vi "PH_Beckhoff_PP_PU.set Ignitron GUI Elements to Default.vi"(0 "i ref in":refnum<vi>, 2 "PUs":T2[](array[typedef]), 5 "error in":errorcluster) -> (14 "i ref out":refnum<vi>, 19 "error out":errorcluster)   [LabVIEW 2014, in "PH_Beckhoff_PP_PU.lvlib"]
uses:
  PH_Beckhoff_PP_PU.lvlib
  PH_PP_Common/PH_PP_Common.PUs.ctl
  PH_Beckhoff_PP_PU.Igni Tags.ctl
  PH_Common/Names/PH_Names.Subsystems.ctl
  PH_PP_Common/PH_PP_Common.Devices.ctl
  PH_Common/PH_Common.lvlib
  PH_PP_Common/PH_PP_Common.lvlib
panel:
  in  "Ignitron Tags":T1
  in  "PU":T2
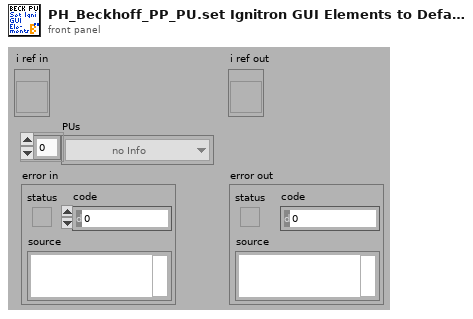
[diagram p1: front panel]
types:
  T1 = typedef "PH_Beckhoff_PP_PU.lvlib/PH_Beckhoff_PP_PU.Igni Tags.ctl" = enum16{"heating-on", "water-on", "Device-on", "Status"}
  T2 = typedef "PH_PP_Common.lvlib/PH_PP_Common.PUs.ctl" = enum16{"no Info", "PA-19mm-1", "PA-19mm-2", "PA-45mm-PILC", "PA-45mm-MAIN", "MA-PU-1", "MA-PU-2", "MA-PU-3", "MA-PU-4", "MA-PU-5", "MA-PU-6", "MA-FR", "MA-PILC", "PA-45mm-DP"}
  T3 = typedef "PH_Common.lvlib/PH_Names.Subsystems.ctl" = enum16{"no Info", "fs-FE", "ns-FE", "PA", "MA", "MAS", "COS", "Exp-LB", "Exp-LL", "PP", "PILS"}
  T4 = typedef "PH_Beckhoff_PP_PU.lvlib/PH_Beckhoff_PP_PU.i attribute.ctl" = cluster{"HV Meas":cluster{"Input GUI Ref":refnum<vi>, "Voltage Service ID":i32, "Voltage [V]":dbl, "Quality":bool, "# in Data":i32}[], "Trigger":cluster{"Status":cluster{"GUI Ref":refnum<vi>, "Status Service ID":i32, "Status":T5}, "last shot:":cluster{"GUI Ref":refnum<vi>, "Service ID":i32, "Time":string}, "DIs":cluster{"triggered":cluster{"GUI Ref":refnum<vi>, "# in Data":i32}, "fired":cluster{"GUI Ref":refnum<vi>, "# in Data":i32}}, "GUI Ref Indicator":refnum<vi>}[], "RR":cluster{"Status":cluster{"GUI Ref":refnum<vi>, "Status Service ID":i32, "Status":T5}, "DIs":cluster{"closed":cluster{"GUI Ref":refnum<vi>, "# in Data":i32}, "open":cluster{"GUI Ref":refnum<vi>, "# in Data":i32}}, "Close":cluster{"GUI Ref":refnum<vi>, "# in Data":i32}, "GUI Ref Indicator":refnum<vi>}[], "Igni":cluster{"Status":cluster{"GUI Ref":refnum<vi>, "Status Service ID":i32, "Status":T5}, "DIs":cluster{"heating on":cluster{"GUI Ref":refnum<vi>, "# in Data":i32}, "water on":cluster{"GUI Ref":refnum<vi>, "# in Data":i32}}, "Device on":cluster{"GUI Ref":refnum<vi>, "# in Data":i32}, "GUI Ref Indicator":refnum<vi>}[], "PSU":cluster{"Status":cluster{"GUI Ref":refnum<vi>, "Status Service ID":i32, "Status":T5}, "Limit Service ID":i32, "DIs":cluster{"inhibit":cluster{"GUI Ref":refnum<vi>, "# in Data":i32}, "end of charge":cluster{"GUI Ref":refnum<vi>, "# in Data":i32}, "HV on":cluster{"GUI Ref":refnum<vi>, "# in Data":i32}, "overtemp":cluster{"GUI Ref":refnum<vi>, "# in Data":i32}, "interlock":cluster{"GUI Ref":refnum<vi>, "# in Data":i32}, "load fault":cluster{"GUI Ref":refnum<vi>, "# in Data":i32}, "sum fault":cluster{"GUI Ref":refnum<vi>, "# in Data":i32}, "HV off":cluster{"GUI Ref":refnum<vi>, "# in Data":i32}, "DC ok":cluster{"GUI Ref":refnum<vi>, "# in Data":i32}}, "AIs":cluster{"voltage":cluster{"GUI Ref":refnum<vi>, "# in Data":i32}, "current":cluster{"GUI Ref":refnum<vi>, "# in Data":i32}}, "DAs":cluster{"inhibit":cluster{"GUI Ref":refnum<vi>, "# in Data":i32}, "interlock":cluster{"GUI Ref":refnum<vi>, "# in Data":i32}, "HV on":cluster{"GUI Ref":refnum<vi>, "# in Data":i32}, "Reset":cluster{"GUI Ref":refnum<vi>, "# in Data":i32}}, "AAs":cluster{"Voltage to set":cluster{"GUI Ref":refnum<vi>, "# in Data":i32}}, "GUI Ref Indicator":refnum<vi>}[], "reconfigured":cluster{"?":bool, "GUI Ref":refnum<vi>}, "PU Rack Type":T6, "HV Meas Info":T7, "PSU Info":T8}
  T5 = typedef "PH_StatusHandler.lvlib/PH_StatusHandler.Status.ctl" = i16
  T6 = typedef "PH_Beckhoff_PP_PU.lvlib/PH_Beckhoff_PP_PU.PU Rack Type.ctl" = enum16{"no Info", "PA 19mm", "PA 45mm", "MA PU 1 and 2", "MA PU 3 and 4", "MA PU 5 and 6", "MA FR and PILC"}
  T7 = typedef "PH_Beckhoff_PP_PU.lvlib/PH_Beckhoff_PP_PU.HV Meas Info.ctl" = cluster{"Period Time [s]":dbl, "Subtractor 1 [Hz]":dbl, "Devider 1 [Hz/kV]":dbl, "Subtractor 2 [Hz]":dbl, "Devider 2 [Hz/kV]":dbl}
  T8 = typedef "PH_Beckhoff_PP_PU.lvlib/PH_Beckhoff_PP_PU.PSU Info.ctl" = cluster{"Limits 1 [V]":cluster{"Lower":dbl, "Upper":dbl}, "Limits 2 [V]":cluster{"Lower":dbl, "Upper":dbl}}
  T9 = cluster{"Status":cluster{"GUI Ref":refnum<vi>, "Status Service ID":i32, "Status":T5}, "DIs":cluster{"heating on":cluster{"GUI Ref":refnum<vi>, "# in Data":i32}, "water on":cluster{"GUI Ref":refnum<vi>, "# in Data":i32}}, "Device on":cluster{"GUI Ref":refnum<vi>, "# in Data":i32}, "GUI Ref Indicator":refnum<vi>}[]
  T10 = typedef "PH_PP_Common.lvlib/PH_PP_Common.Devices.ctl" = enum16{"no Info", "Igni", "RR", "DumpRoss", "PSU", "Trigger", "HV-Meas", "Rods", "Chiller", "Conductivity", "Mercury"}
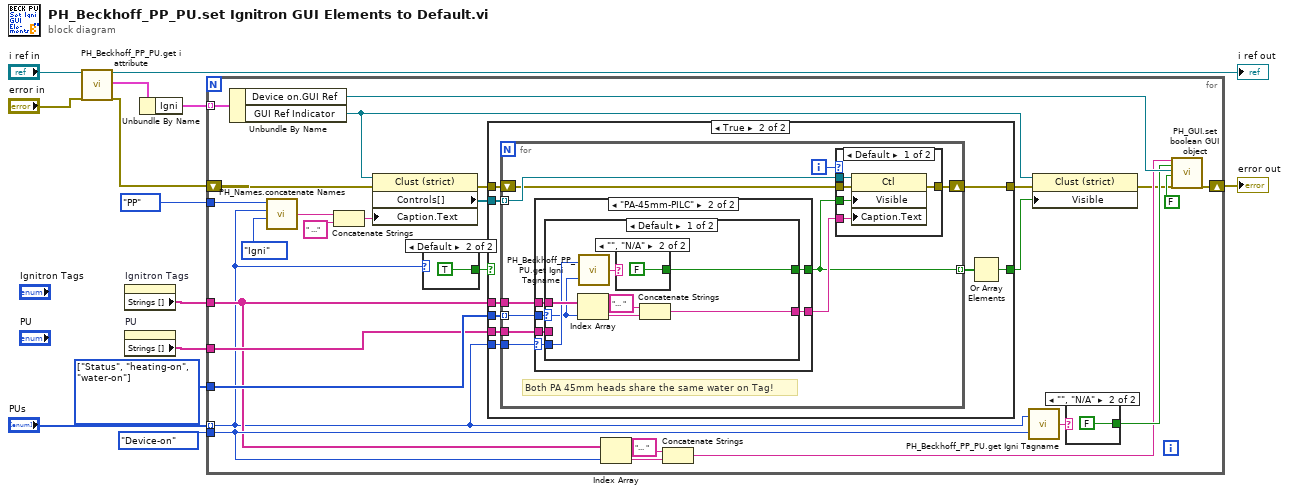
[diagram p0: block diagram]
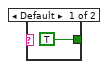
[diagram p2: hidden frame]
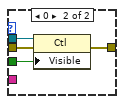
[diagram p4: hidden frame]
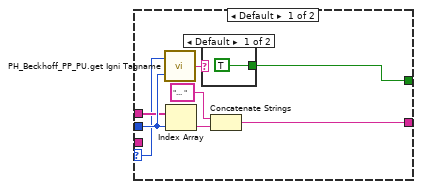
[diagram p5: hidden frame]
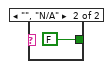
[diagram p6: hidden frame]
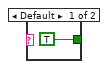
[diagram p7: hidden frame]
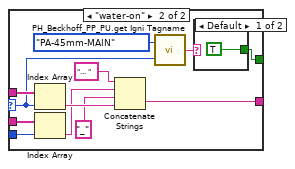
[diagram p8: hidden frame]
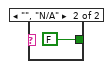
[diagram p9: hidden frame]
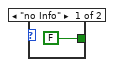
[diagram p10: hidden frame]
diagram:
  w2 = T1[] [enum."Status", enum."heating-on", enum."water-on"] items=["heating-on", "water-on", "Device-on", "Status"]
  n1 = call "PH_Beckhoff_PP_PU.get i attribute.vi"("i ref in"="i ref in", "error in (no error)"="error in") -> ("i ref out"=→"i ref out":refnum<vi>, "i attribute"=w10:T4, "error out"=w8:errorcluster)  [unwired: 15 in]
  n2 = property on="Ignitron Tags" class="Enum (strict)"() -> ("Strings []"=w3:string[])  [unwired: 2 in, 2 out]
  n3 = property on="PU" class="Enum (strict)"() -> ("Strings []"=w11:string[])  [unwired: 2 in, 2 out]
  n4 = Unbundle By Name(w10) -> ("Igni"=w9:T9)
  n5 = for {
    tunnel: w9 -> [w40] mode=indexing
    shift-right: [w32] -> w12
    shift-left: w8 -> [w38]
    tunnel: "PUs" -> [w21] mode=indexing
    tunnel: w2 -> [w37]
    tunnel: w11 -> [w26]
    tunnel: w3 -> [w22]
    tunnel: PH_Beckhoff_PP_PU.Igni_Tags."Device-on" ("Igni Tag") -> [w25]
    tunnel: PH_Names.Subsystems."PP" ("Subsystem") -> [w19]
    n6 = Unbundle By Name(w40) -> ("Device on.GUI Ref"=w31:refnum<vi>, "GUI Ref Indicator"=w15:refnum<vi>)
    n7 = call "PH_Names.concatenate Names.vi"("Devices (no info)"=PH_PP_Common.Devices."Igni", "PU (no info)"=w21, "Subsystem"=w19) -> ("Subsystem_PU_Devices_Comm Type"=w20:string)  [unwired: 1 in]
    n8 = Concatenate Strings(w20, " ..." ("string")) -> (w34:string)
    n9 = property class="Clust (strict)"(reference=w15, error in=w38, "Caption.Text"=w34) -> (error out=w39:errorcluster, "Controls[]"=w35:refnum<vi>[])  [unwired: 1 out]
    n10 = case shown="Default" w21 {
      tunnel: [FALSE TRUE] -> w36
      frame "no Info" {
      }
      frame Default {
      }
    }
    n11 = case shown="True" w36 {
      selector: w36 -> [w43 _]
      tunnel: w35 -> [_ w53]
      tunnel: w39 -> [w44 w52]
      tunnel: [w44 w51] -> w16
      tunnel: w37 -> [_ w50]
      tunnel: w21 -> [_ w49]
      tunnel: w22 -> [_ w48]
      tunnel: w26 -> [_ w47]
      tunnel: [w43 w45] -> w14
      frame False {
      }
      frame True {
        n12 = for {
          tunnel: w53 -> [w56] mode=indexing
          shift-right: [w59] -> w51
          shift-left: w52 -> [w55]
          tunnel: w49 -> [w61]
          tunnel: w50 -> [w63] mode=indexing
          tunnel: w48 -> [w62]
          tunnel: w47 -> [w60]
          tunnel: [w54] -> w46 mode=indexing
          i -> [w57]
          # "Both PA 45mm heads share the same water on Tag!"
          n13 = case shown="\"PA-45mm-PILC\"" w61 {
            selector: w61 -> [w75 w87]
            tunnel: w63 -> [w80 w86]
            tunnel: w62 -> [w79 w88]
            tunnel: w60 -> [_ w85]
            tunnel: [w73 w84] -> w54
            tunnel: [w74 w83] -> w58
            frame Default {
              n14 = call "PH_Beckhoff_PP_PU.get Igni Tagname.vi"("Igni Tag"=w80, "PU"=w75) -> ("Igni Tagname"=w78:string)
              n15 = Index Array(array=w79, index=w80) -> (element=w77:string)
              n16 = case shown="Default" w78 {
                tunnel: [TRUE FALSE] -> w73
                frame Default {
                }
                frame "", "N/A" {
                }
              }
              n17 = Concatenate Strings("... " ("string"), w77) -> (w74:string)
            }
            frame "PA-45mm-PILC" {
              n18 = case shown="Default" w86 {
                selector: w86 -> [w91 w107]
                tunnel: w88 -> [w96 w110]
                tunnel: w87 -> [w92 w102]
                tunnel: w85 -> [_ w101]
                tunnel: [w89 w99] -> w83
                tunnel: [w90 w100] -> w84
                frame Default {
                  n19 = Index Array(array=w96, index=w91) -> (element=w94:string)
                  n20 = call "PH_Beckhoff_PP_PU.get Igni Tagname.vi"("Igni Tag"=w91, "PU"=w92) -> ("Igni Tagname"=w95:string)
                  n21 = case shown="\"\", \"N/A\"" w95 {
                    tunnel: [TRUE FALSE] -> w90
                    frame Default {
                    }
                    frame "", "N/A" {
                    }
                  }
                  n22 = Concatenate Strings("... " ("string"), w94) -> (w89:string)
                }
                frame "water-on" {
                  n23 = Index Array(array=w110, index=w107) -> (element=w108:string)
                  n24 = Index Array(array=w101, index=w102) -> (element=w104:string)
                  n25 = Concatenate Strings("... " ("string"), w104, "_" ("string"), w108) -> (w99:string)
                  n26 = call "PH_Beckhoff_PP_PU.get Igni Tagname.vi"("Igni Tag"=w107, "PU"=PH_PP_Common.PUs."PA-45mm-MAIN") -> ("Igni Tagname"=w109:string)
                  n27 = case shown="Default" w109 {
                    tunnel: [TRUE FALSE] -> w100
                    frame Default {
                    }
                    frame "", "N/A" {
                    }
                  }
                }
              }
            }
          }
          n28 = case shown="Default" w57 {
            tunnel: w55 -> [w68 w72]
            tunnel: [w67 w71] -> w59
            tunnel: w54 -> [w66 w70]
            tunnel: w56 -> [w65 w69]
            tunnel: w58 -> [w64 _]
            frame Default {
              n29 = property class="Ctl"(reference=w65, error in=w68, "Visible"=w66, "Caption.Text"=w64) -> (error out=w67:errorcluster)  [unwired: 1 out]
            }
            frame 0 {
              n30 = property class="Ctl"(reference=w69, error in=w72, "Visible"=w70) -> (error out=w71:errorcluster)  [unwired: 1 out]
            }
          }
        }
        n31 = Or Array Elements(Boolean array=w46) -> (logical OR=w45:bool)
      }
    }
    n32 = Index Array(array=w22, index=w25) -> (element=w27:string)
    n33 = Concatenate Strings("... " ("string"), w27) -> (w24:string)
    n34 = call "PH_Beckhoff_PP_PU.get Igni Tagname.vi"("Igni Tag"=w25, "PU"=w21) -> ("Igni Tagname"=w29:string)
    n35 = property class="Clust (strict)"(reference=w15, error in=w16, "Visible"=w14) -> (error out=w17:errorcluster)  [unwired: 1 out]
    n36 = case shown="\"\", \"N/A\"" w29 {
      tunnel: [TRUE FALSE] -> w28
      frame Default {
      }
      frame "", "N/A" {
      }
    }
    n37 = call "PH_GUI.set boolean GUI object.vi"("Caption"=w24, "Visible (true)"=w28, "Boolean Knob GUI Ref"=w31, "Value"=FALSE, "error in (no error)"=w17) -> ("error out"=w32:errorcluster)  [unwired: 14 in]
  }
  "error out" <- w12
